vi "Save Log.vi"(10 "Array":string[](array[string]), 11 "VI in":refnum<vi>) -> ()   [LabVIEW 2013, in "main.lvlib"]
uses:
  main.lvlib
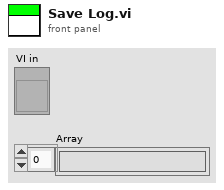
[diagram p1: front panel]
types:
  T1 = enum16{"open", "replace", "create", "open or create", "replace or create", "replace or create with confirmation"}
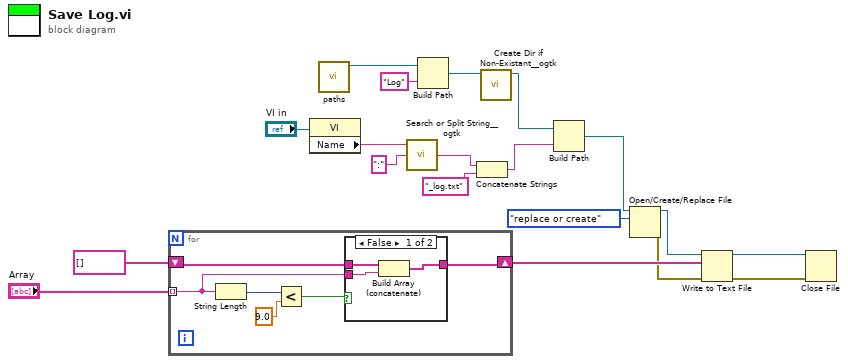
[diagram p0: block diagram]
diagram:
  n1 = for {
    tunnel: "Array" -> [w22] mode=indexing
    shift-right: [w24] -> w16
    shift-left: string[] [] -> [w23]
    n2 = String Length(string=w22) -> (length=w20:i32)
    n3 = Less?(x=w20, y=9.0) -> (x < y?=w25:bool)
    n4 = case shown="False" w25 {
      tunnel: [w28 w29] -> w24
      tunnel: w23 -> [w27 w29]
      tunnel: w22 -> [w26 _]
      frame False {
        n5 = Build Array (concatenate)(w27, w26) -> (w28:string[])
      }
      frame True {
      }
    }
  }
  n6 = property class="VI"(reference="VI in") -> ("Name"=w15:string)  [unwired: 1 in, 2 out]
  n7 = call "paths.vi"() -> ("PubAppData"=w10:path)  [unwired: 8 in, 3 out]
  n8 = call <userlib>:"Search or Split String__ogtk.vi"("search string/char (-)"=":", "string"=w15) -> ("substring after match"=w13:string)  [unwired: 1 in, 2 out]
  n9 = Build Path(base path=w10, name or relative path="Log") -> (appended path=w2:path)
  n10 = Concatenate Strings(w13, "_log.txt" ("string")) -> (w11:string)
  n11 = call <userlib>:"Create Dir if Non-Existant__ogtk.vi"("Directory Path"=w2) -> ("dup Directory Path"=w1:path)  [unwired: 8 in, 2 out]
  n12 = Build Path(base path=w1, name or relative path=w11) -> (appended path=w8:path)
  n13 = Open/Create/Replace File(file path (use dialog)=w8, operation (0:open)=T1."replace or create") -> (refnum out=w7:refnum<file>, error out=w3:errorcluster)  [unwired: 4 in, 1 out]
  n14 = Write to Text File(file (use dialog)=w7, text=w16, error in=w3) -> (refnum out=w5:refnum<file>, error out=w4:errorcluster)  [unwired: 1 in, 1 out]
  n15 = Close File(refnum=w5, error in=w4) -> ()  [unwired: 2 out]
